vi "Read App DAQ Settings File--0.vi"(8 "error in (no error)":errorcluster, 11 "SettingsFolder":path) -> (0 "error out":errorcluster, 1 "default file created":bool, 2 "Configuration":T3, 3 "Settings Folder out":path)   [LabVIEW 2017]
doc: "Reads file: \"IOConfig.ini\" at \"ConfigFolder\" folder."
uses:
  <vilib>/Utility/config.llb/NI_LVConfig.lvlib
  <userlib>/_OpenG.lib/file/file.llb/File Exists - Scalar__ogtk.vi
  DataTypes/TD AI InstSettings--cluster.ctl
  Process/ProcessSupport/TD SimAI Ranges--cluster.ctl
panel:
  # "NOTE: This utility is only used during development\nfor debugging DAQ class."
  # "Reads file: \"Settings.ini\"\nat \"SettingsFolder\" folder."
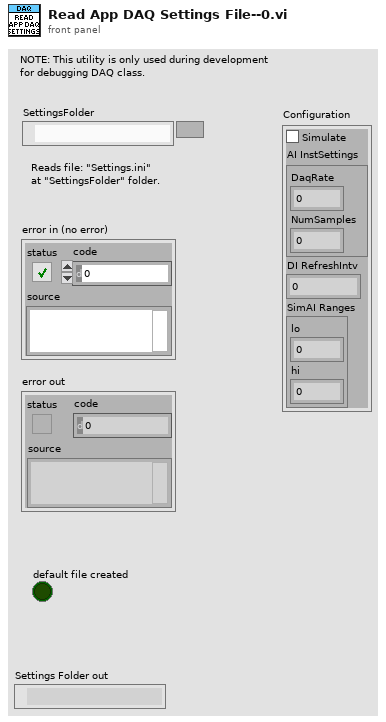
[diagram p1: front panel]
types:
  T1 = typedef "DAQ.lvclass/TD AI InstSettings--cluster.ctl" = cluster{"DaqRate":dbl, "NumSamples":i32}
  T2 = typedef "DAQ.lvclass/TD SimAI Ranges--cluster.ctl" = cluster{"lo":dbl, "hi":dbl}
  T3 = cluster{"Simulate":bool, "AI InstSettings":T1, "DI RefreshIntv":i32, "SimAI Ranges":T2}
  T4 = typedef "NI_LVConfig.lvlib/Config Data RefNum.ctl" = refnum<k1>
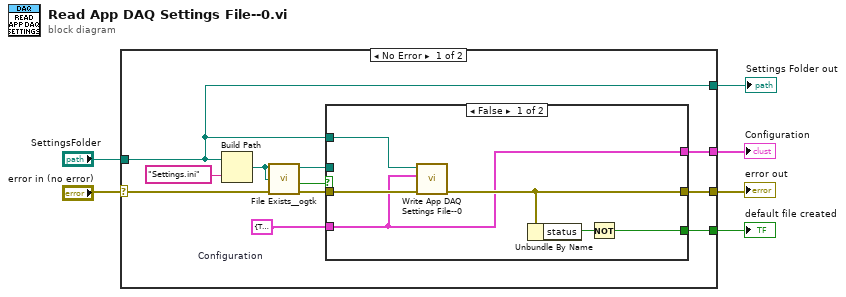
[diagram p0: block diagram]
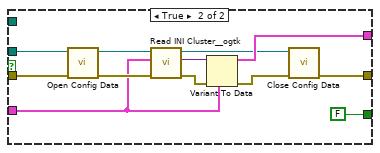
[diagram p2: hidden frame]
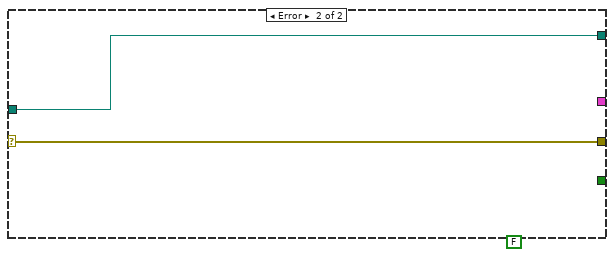
[diagram p3: hidden frame]
diagram:
  n1 = case shown="No Error" "error in (no error)" {
    selector: "error in (no error)" -> [w13 w35]
    tunnel: "SettingsFolder" -> [w8 w34]
    tunnel: [w15 _] -> w5
    tunnel: [w14 w35] -> w4
    tunnel: [w9 _] -> w2
    tunnel: [w8 w34] -> w1
    frame No Error {
      w7 = T3 {"Simulate"=TRUE, "AI InstSettings"={"DaqRate"=1000.0, "NumSamples"=200}, "DI RefreshIntv"=100, "SimAI Ranges"={"lo"=0.0, "hi"=10.0}}  # Configuration
      n2 = Build Path(base path=w8, name or relative path="Settings.ini") -> (appended path=w11:path)
      n3 = call-poly <userlib>:"File Exists__ogtk.vi"("file path"=w11) -> ("exists"=w10:bool)  [unwired: 6 in, 1 out]
      n4 = case shown="False" w10 {
        tunnel: w11 -> [_ w33]
        tunnel: [w16 w32] -> w15
        tunnel: [w19 w31] -> w14
        tunnel: w13 -> [w21 w24]
        tunnel: w8 -> [w20 _]
        tunnel: w7 -> [w16 w23]
        tunnel: [w17 FALSE] -> w9
        frame False {
          n5 = call "Write App DAQ Settings File--0.vi"("error in (no error)"=w21, "Configuration"=w16, "SettingsFolder"=w20) -> ("error out"=w19:errorcluster)  [unwired: 7 in, 1 out]
          n6 = Unbundle By Name(w19) -> ("status"=w18:bool)
          n7 = Not(x=w18) -> (.not. x?=w17:bool)
        }
        frame True {
          n8 = call <vilib>:"Open Config Data.vi"("error in (no error)"=w24, "configuration file path"=w33) -> ("error out"=w29:errorcluster, "refnum"=w30:T4)  [unwired: 7 in, 1 out]
          n9 = call <userlib>:"Read INI Cluster__ogtk.vi"("error in (no error)"=w29, "INI Fomatted Cluster Type"=w23, "refnum"=w30) -> ("error out"=w27:errorcluster, "INI Fomatted Cluster"=w25:variant, "dup refnum"=w28:T4)  [unwired: 4 in, 2 out]
          n10 = Variant To Data(error in=w27, type=w23, Variant=w25) -> (data=w32:T3, error out=w26:errorcluster)
          n11 = call <vilib>:"Close Config Data.vi"("error in (no error)"=w26, "refnum"=w28) -> ("error out"=w31:errorcluster)  [unwired: 8 in, 1 out]
        }
      }
    }
    frame Error {
      (unwired) FALSE ("cancelled")
    }
  }
  "Configuration" <- w5
  "error out" <- w4
  "default file created" <- w2
  "Settings Folder out" <- w1
